vi "Delay_region_sample_control_v3.vi"(4 "K2":dbl=0.4, 5 "K1":dbl=0.4, 6 "Z":dbl, 7 "X":dbl, 8 "Beta":dbl, 9 "Alpha":dbl) -> (1 "delta_T":dbl, 2 "delta_X":dbl, 3 "delta_Z":dbl)   [LabVIEW 2009]
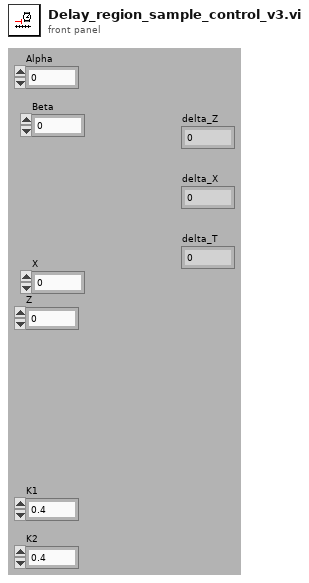
[diagram p1: front panel]
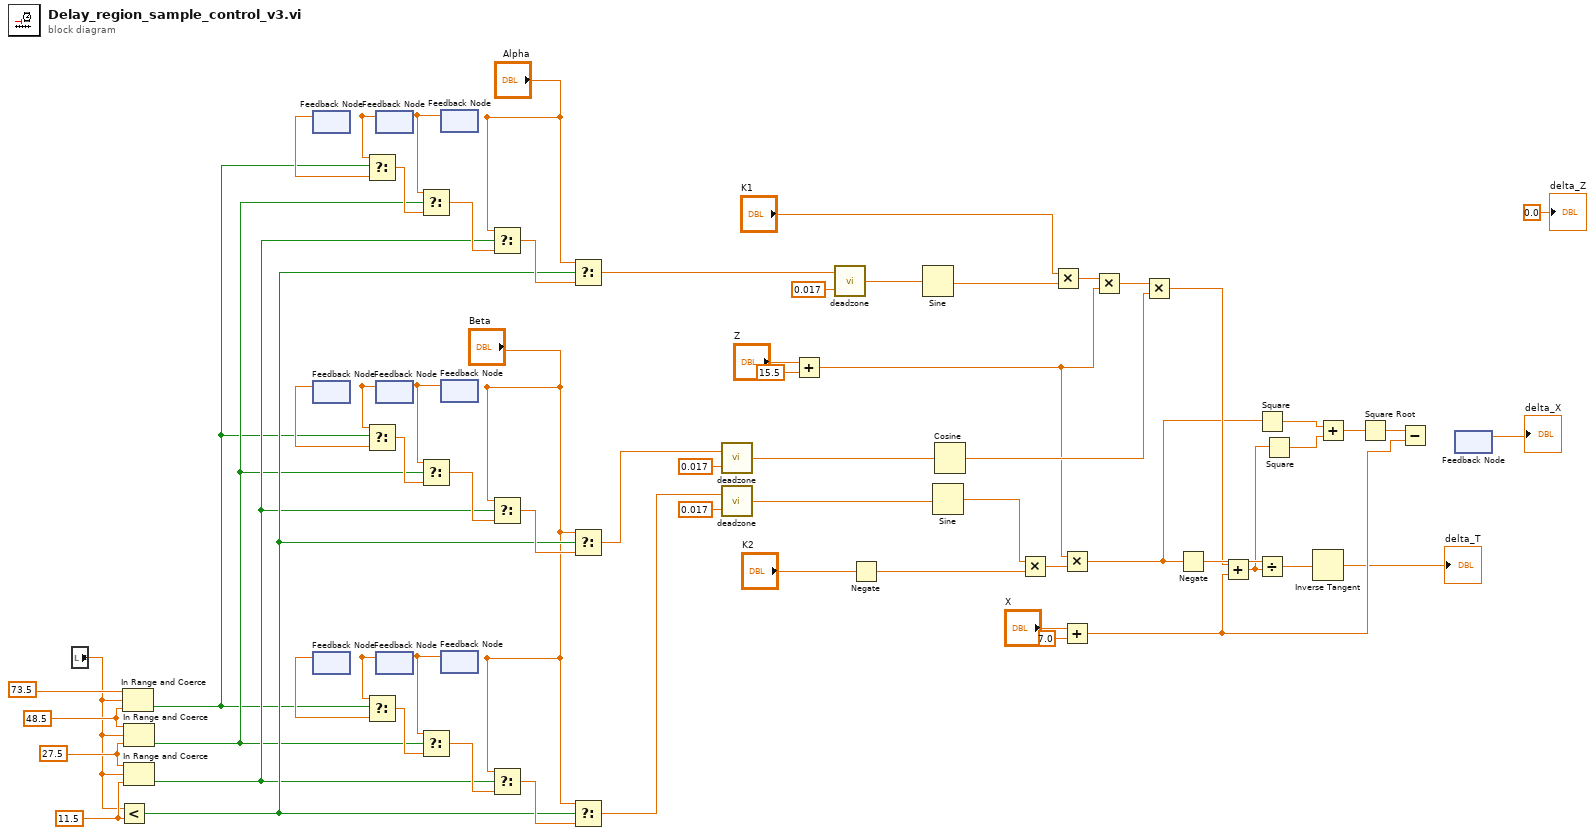
[diagram p0: block diagram]
diagram:
  w11 = 48.5 ("y")
  w10 = 27.5 ("y")
  w9 = 11.5 ("y")
  n1 = local read "Z"() -> (w4:dbl)
  n2 = Less?(x=w4, y=w9) -> (x < y?=w8:bool)
  n3 = In Range and Coerce(upper limit=73.5 ("y"), x=w4, lower limit=w11) -> (In Range?=w5:bool)  [unwired: 1 out]
  n4 = In Range and Coerce(upper limit=w11, x=w4, lower limit=w10) -> (In Range?=w6:bool)  [unwired: 1 out]
  n5 = In Range and Coerce(upper limit=w10, x=w4, lower limit=w9) -> (In Range?=w7:bool)  [unwired: 1 out]
  n6 = feedback #1() -> (w29:dbl)  [unwired: 1 in]
  n7 = feedback #2() -> (w23:dbl)  [unwired: 1 in]
  n8 = feedback #3() -> (w16:dbl)  [unwired: 1 in]
  n9 = feedback #4() -> (w27:dbl)  [unwired: 1 in]
  n10 = Select(t=w27, s=w5, f=w29) -> (s? t:f=w30:dbl)
  n11 = feedback #5() -> (w21:dbl)  [unwired: 1 in]
  n12 = Select(t=w21, s=w5, f=w23) -> (s? t:f=w24:dbl)
  n13 = feedback #6() -> (w14:dbl)  [unwired: 1 in]
  n14 = Select(t=w14, s=w5, f=w16) -> (s? t:f=w17:dbl)
  n15 = feedback #7() -> (w28:dbl)  [unwired: 1 in]
  n16 = Select(t=w28, s=w6, f=w30) -> (s? t:f=w34:dbl)
  n17 = feedback #8() -> (w22:dbl)  [unwired: 1 in]
  n18 = Select(t=w22, s=w6, f=w24) -> (s? t:f=w25:dbl)
  n19 = feedback #9() -> (w15:dbl)  [unwired: 1 in]
  n20 = Select(t=w15, s=w6, f=w17) -> (s? t:f=w18:dbl)
  n21 = Select(t="Alpha", s=w7, f=w34) -> (s? t:f=w35:dbl)
  n22 = Select(t="Beta", s=w7, f=w25) -> (s? t:f=w26:dbl)
  n23 = Select(t="Beta", s=w7, f=w18) -> (s? t:f=w19:dbl)
  n24 = Select(t="Alpha", s=w8, f=w35) -> (s? t:f=w33:dbl)
  n25 = Select(t="Beta", s=w8, f=w26) -> (s? t:f=w20:dbl)
  n26 = Select(t="Beta", s=w8, f=w19) -> (s? t:f=w13:dbl)
  n27 = call "deadzone.vi"("threshold"=0.017, "in"=w20) -> ("out"=w38:dbl)
  n28 = call "deadzone.vi"("threshold"=0.017, "in"=w13) -> ("out"=w32:dbl)
  n29 = Add(x="Z", y=15.5) -> (x+y=w55:dbl)
  n30 = call "deadzone.vi"("threshold"=0.017, "in"=w33) -> ("out"=w39:dbl)
  n31 = Negate(x="K2") -> (-x=w40:dbl)
  n32 = Sine(x=w39) -> (sin(x)=w61:dbl)
  n33 = Sine(x=w32) -> (sin(x)=w57:dbl)
  n34 = Cosine(x=w38) -> (cos(x)=w58:dbl)
  n35 = Multiply(x=w57, y=w40) -> (x*y=w56:dbl)
  n36 = Multiply(x="K1", y=w61) -> (x*y=w60:dbl)
  n37 = Multiply(x=w55, y=w56) -> (x*y=w51:dbl)
  n38 = Add(x="X", y=7.0) -> (x+y=w45:dbl)
  n39 = Multiply(x=w60, y=w55) -> (x*y=w59:dbl)
  n40 = Multiply(x=w59, y=w58) -> (x*y=w53:dbl)
  n41 = Negate(x=w51) -> (-x=w54:dbl)
  n42 = Add(x=w53, y=w45) -> (x+y=w50:dbl)
  n43 = Square(x=w51) -> (x^2=w49:dbl)
  n44 = Divide(x=w54, y=w50) -> (x/y=w52:dbl)
  n45 = Square(x=w50) -> (x^2=w48:dbl)
  n46 = Inverse Tangent(1:w52) -> (0:→"delta_T":dbl)
  n47 = Add(x=w49, y=w48) -> (x+y=w47:dbl)
  n48 = Square Root(x=w47) -> (sqrt(x)=w46:dbl)
  n49 = Subtract(x=w46, y=w45) -> (x-y=w37:dbl)
  n50 = feedback #10() -> (→"delta_X":dbl)  [unwired: 1 in]
  "delta_Z" <- 0.0 ("delta_Z")
